vi "Add_Pitot_Vel.vi"(1 "Channels from Client In":string[][](array[string])=[["Data Base:Measurement:Type", "LDA & Cw"], ["Data Base:Position:No of Inst", "2"], ["Data Base:Position:X1", "-60"], ["Data Base:Position:X2", ""], ["Data Base:Position:Y1", "2"], ["Data Base:Position:Y2", "0.00"], ["Data Base:Position:Z1", "0.00"], ["Data Base:Position:Z2", "2.00"]]) -> (0 "Channels from Client Out":string[][](array[string])=[["Data Base:Measurement:Type", "LDA & Cw"], ["Data Base:Position:No of Inst", "2"], ["Data Base:Position:X1", "-60"], ["Data Base:Position:X2", ""], ["Data Base:Position:Y1", "2"], ["Data Base:Position:Y2", "0.00"], ["Data Base:Position:Z1", "0.00"], ["Data Base:Position:Z2", "2.00"]])   [LabVIEW 2010]
uses:
  Globals/Meas_global.vi
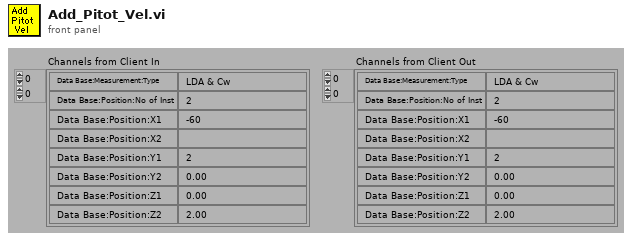
[diagram p1: front panel]
types:
  T1 = typedef "Velocity_cluster.ctl" = cluster{"Name":string, "U":dbl, "u^2":dbl, "u^3/(u^2)^(1.5)":dbl, "u^4/(u^2)^2 -3":dbl, "% u'/U":dbl, "Mean % Err":dbl, "u^4":dbl}
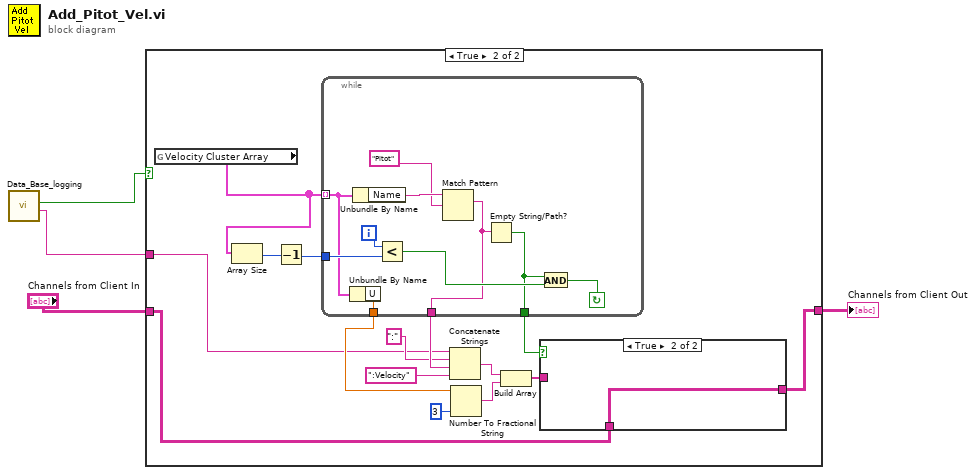
[diagram p0: block diagram]
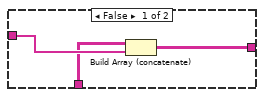
[diagram p3: hidden frame]
diagram:
  n1 = call "Data_Base_logging.vi"() -> ("Close Loop with Pitot?"=w2:bool, "Rig Name"=w1:string)  [unwired: 3 out]
  n2 = case shown="True" w2 {
    tunnel: "Channels from Client In" -> [w5 w8]
    tunnel: [w5 w7] -> w3
    tunnel: w1 -> [_ w6]
    frame False {
    }
    frame True {
      n3 = global read "Meas_global.vi" "Velocity Cluster Array"() -> (w20:T1[])
      n4 = Array Size(array=w20) -> (size(s)=w19:i32)
      n5 = Decrement(x=w19) -> (x-1=w18:i32)
      n6 = while {
        tunnel: [w21] -> w13
        tunnel: [w22] -> w16
        tunnel: [w24] -> w17
        tunnel: w18 -> [w29]
        tunnel: w20 -> [w25] mode=indexing
        i -> [w30]
        stop <- w26 continue-if-true
        n7 = Unbundle By Name(w25) -> ("U"=w21:dbl)
        n8 = Unbundle By Name(w25) -> ("Name"=w28:string)
        n9 = Less?(x=w30, y=w29) -> (x < y?=w27:bool)
        n10 = Match Pattern(string=w28, regular expression="Pitot") -> (match substring=w22:string)  [unwired: 4 out]
        n11 = Empty String/Path?(string/path=w22) -> (empty?=w24:bool)
        n12 = And(x=w24, y=w27) -> (x .and. y?=w26:bool)
      }
      n13 = Concatenate Strings(w6, ":" ("Substring"), w16, ":Velocity" ("Substring")) -> (w11:string)
      n14 = Number To Fractional String(number=w13, precision (6)=i16 3) -> (F-format string=w10:string)  [unwired: 2 out]
      n15 = Build Array(w11, w10) -> (w9:string[])
      n16 = case shown="True" w17 {
        tunnel: w9 -> [w33 _]
        tunnel: w8 -> [w32 w34]
        tunnel: [w31 w34] -> w7
        frame False {
          n17 = Build Array (concatenate)(w32, w33) -> (w31:string[][])
        }
        frame True {
        }
      }
    }
  }
  "Channels from Client Out" <- w3
